vi "WPI_AnalogTriggerOpen.vi"(6 "Filter":bool, 7 "Averaged":bool, 8 "error in (no error)":errorcluster, 9 "LowerLimit (v)":dbl, 10 "UpperLimit (v)":dbl, 11 "AnalogTriggerSource":T1={"DevStatus"={"status"=FALSE, "code"=0, "source"=""}, "Analog Channel"=enum."Invalid"}) -> (0 "error out":errorcluster, 3 "AnalogTriggerDevRef":T3={"DevStatus"={"status"=FALSE, "code"=0, "source"=""}, "AnalogTriggerIndex"=enum."Invalid"})   [LabVIEW 2017]
doc: "Opens and configures a reference to the analog trigger. You must open a reference before using any other AnalogTrigger VIs.\n\nThis software is licensed. Open the labview\\readme\\WPI Robotics Library Open Source License.txt file for more information."
uses:
  <vilib>/Rock Robotics/SystemInterfaces/AnalogTrigger/FPGA_AnalogTriggerDevRef.ctl
  <vilib>/Rock Robotics/SystemInterfaces/AnalogTrigger/FPGA_AnalogTriggerIndex.ctl
  <vilib>/Rock Robotics/WPI/AnalogChannel/WPI_AnalogChannelDevRef.ctl
  <vilib>/Rock Robotics/SystemInterfaces/AI/FPGA_AIChannel.ctl
  <vilib>/Rock Robotics/SystemInterfaces/AnalogTrigger/FPGA_AnalogTriggerSource.ctl
  <vilib>/Rock Robotics/SystemInterfaces/NetworkCommunication/NetComm_UsageReport_ResourceType.ctl
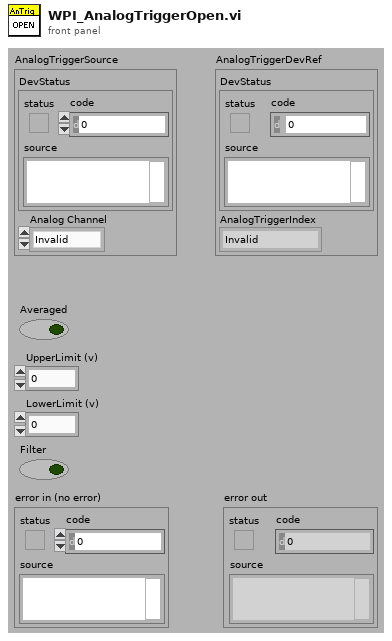
[diagram p1: front panel]
types:
  T1 = typedef "WPI_AnalogChannelDevRef.ctl" = cluster{"DevStatus":errorcluster, "Analog Channel":T2}
  T2 = typedef "FPGA_AIChannel.ctl" = enum8{"AI 0", "AI 1", "AI 2", "AI 3", "AI MXP 0", "AI MXP 1", "AI MXP 2", "AI MXP 3", "Invalid"}
  T3 = typedef "FPGA_AnalogTriggerDevRef.ctl" = cluster{"DevStatus":errorcluster, "AnalogTriggerIndex":T4}
  T4 = typedef "FPGA_AnalogTriggerIndex.ctl" = enum8{"Trig 0", "Trig 1", "Trig 2", "Trig 3", "Trig 4", "Trig 5", "Trig 6", "Trig 7", "Invalid"}
  T5 = typedef "NetComm_UsageReport_ResourceType.ctl" = enum8{"Controller", "Module", "Language", "CANPlugin", "Accelerometer", "ADXL345", "AnalogChannel", "AnalogTrigger", "AnalogTriggerOutput", "CANJaguar", "Compressor", "Counter", "Dashboard", "DigitalInput", "DigitalOutput", "DriverStationCIO", "DriverStationEIO", "DriverStationLCD", "Encoder", "GearTooth", "Gyro", "I2C", "Framework", "Jaguar", "Joystick", "Kinect", "KinectStick", "PIDController", "Preferences", "PWM", "Relay", "RobotDrive", "SerialPort", "Servo", "Solenoid", "SPI", "Task", "Ultrasonic", "Victor", "Button", "Command", "AxisCamera", "PCVideoServer", "SmartDashboard", "Talon", "HiTechnicColorSensor", "HiTechnicAccel", "HiTechnicCompass", "SRF08", "AnalogOutput", "Victor SP", "Talon SRX", "CAN Talon SRX", "ADXL362 Accel", "ADXRS450 Gyro", "Rev SPARK", "Mindsensors SD540", "Digital Filter", "ADIS16448", "PDP", "PCM", "PigeonIMU", "Nidec Brushless", "CTRE CANifier", "CTRE Future 0", "CTRE Future 1", "CTRE Future 2", "CTRE Future 3", "CTRE Future 4", "CTRE Future 5", "CTRE Future 6"}
  T6 = typedef "FPGA_AnalogTriggerSource.ctl" = cluster{"Channel":T2, "Averaged":bool, "Filter":bool}
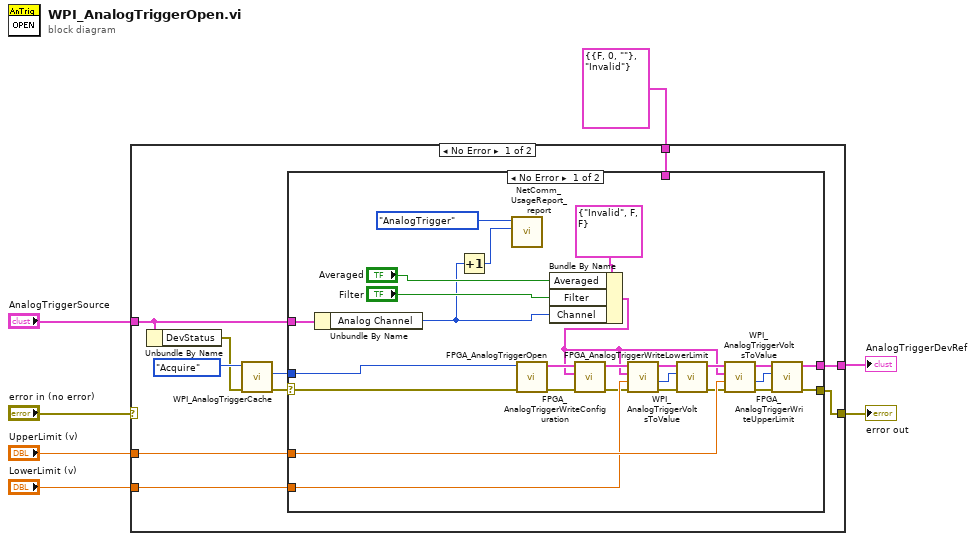
[diagram p0: block diagram]
diagram:
  n1 = case shown="No Error" "error in (no error)" {
    selector: "error in (no error)" -> [_ w46]
    tunnel: "AnalogTriggerSource" -> [w8 _]
    tunnel: [w14 w47] -> w3
    tunnel: [w13 w46] -> w5
    tunnel: T3 {"DevStatus"={"status"=FALSE, "code"=0, "source"=""}, "AnalogTriggerIndex"=enum."Invalid"} ("AnalogTriggerDevRef") -> [w12 w47]
    tunnel: "UpperLimit (v)" -> [w11 _]
    tunnel: "LowerLimit (v)" -> [w10 _]
    frame No Error {
      n2 = Unbundle By Name(w8) -> ("DevStatus"=w9:errorcluster)
      n3 = call <vilib>:"WPI_AnalogTriggerCache.vi"("error in (no error)"=w9, "Operation"=enum16{"Acquire", "Release"}."Acquire") -> ("error out"=w17:errorcluster, "AnalogTriggerAllocated"=w15:T4)  [unwired: 1 in, 7 out]
      n4 = case shown="No Error" w17 {
        selector: w17 -> [w43 w44]
        tunnel: w15 -> [w42 _]
        tunnel: w8 -> [w39 _]
        tunnel: [w34 w45] -> w14
        tunnel: [w29 w44] -> w13
        tunnel: w12 -> [_ w45]
        tunnel: w11 -> [w38 _]
        tunnel: w10 -> [w30 _]
        frame No Error {
          n5 = Unbundle By Name(w39) -> ("Analog Channel"=w24:T2)
          n6 = Increment(x=w24) -> (x+1=w25:T2)
          n7 = call <vilib>:"NetComm_UsageReport_report.vi"("Instance Number"=w25, "Resource Type"=NetComm_UsageReport_ResourceType."AnalogTrigger") -> ()  [unwired: 10 in]
          n8 = call <vilib>:"FPGA_AnalogTriggerOpen.vi"("error in"=w43, "AnalogTriggerChannel"=w42) -> ("error out"=w23:errorcluster, "AnalogTriggerDevRef"=w35:T3)  [unwired: 1 in, 7 out]
          n9 = Bundle By Name(cluster=T6 {"Channel"=enum."Invalid", "Averaged"=FALSE, "Filter"=FALSE} ("AnalogTriggerSource"), "Averaged"="Averaged", "Filter"="Filter", "Channel"=w24) -> (w18:T6)
          n10 = call <vilib>:"FPGA_AnalogTriggerWriteConfiguration.vi"("error in (no error)"=w23, "AnalogTriggerSource"=w18, "AnalogTriggerDevRef"=w35) -> ("error out"=w22:errorcluster, "AnalogTriggerDevRef"=w33:T3)  [unwired: 7 out]
          n11 = call <vilib>:"WPI_AnalogTriggerVoltsToValue.vi"("error in (no error)"=w22, "Voltage"=w30, "AnalogTriggerSource"=w18, "AnalogTriggerDevRef"=w33) -> ("error out"=w21:errorcluster, "Value"=w31:i32, "AnalogTriggerDevRef"=w32:T3)  [unwired: 1 in, 4 out]
          n12 = call <vilib>:"FPGA_AnalogTriggerWriteLowerLimit.vi"("error in (no error)"=w21, "LowerLimit"=w31, "AnalogTriggerDevRef"=w32) -> ("error out"=w20:errorcluster, "AnalogTriggerDevRef"=w28:T3)  [unwired: 7 out]
          n13 = call <vilib>:"WPI_AnalogTriggerVoltsToValue.vi"("error in (no error)"=w20, "Voltage"=w38, "AnalogTriggerSource"=w18, "AnalogTriggerDevRef"=w28) -> ("error out"=w19:errorcluster, "Value"=w37:i32, "AnalogTriggerDevRef"=w27:T3)  [unwired: 1 in, 4 out]
          n14 = call <vilib>:"FPGA_AnalogTriggerWriteUpperLimit.vi"("error in (no error)"=w19, "UpperLimit"=w37, "AnalogTriggerDevRef"=w27) -> ("error out"=w29:errorcluster, "AnalogTriggerDevRef"=w34:T3)  [unwired: 7 out]
        }
        frame Error {
        }
      }
    }
    frame Error {
    }
  }
  "AnalogTriggerDevRef" <- w3
  "error out" <- w5
